vi "First Event Structure.vi"() -> ()   [LabVIEW 2015]
panel:
  out "Boolean":bool
  out "current time":timestamp
  in  "Stop":bool
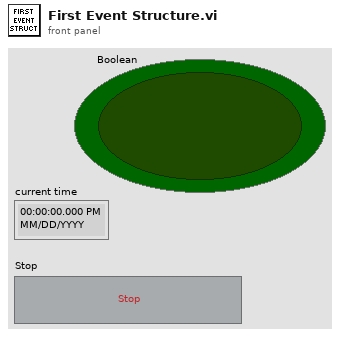
[diagram p1: front panel]
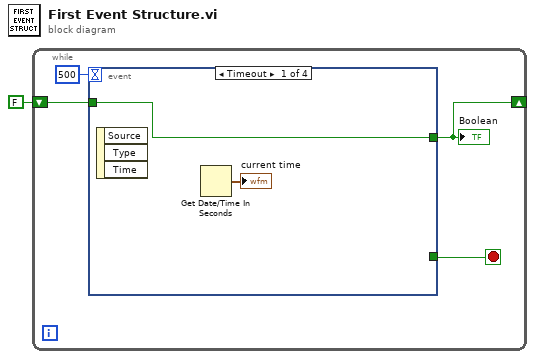
[diagram p0: block diagram]
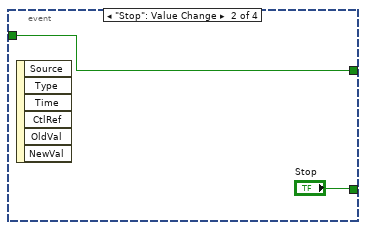
[diagram p2: hidden frame]
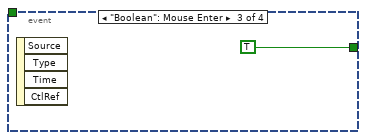
[diagram p3: hidden frame]
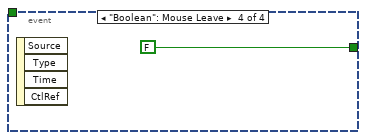
[diagram p4: hidden frame]
diagram:
  n1 = while {
    shift-right: [w3] -> _
    shift-left: FALSE ("Boolean") -> [w2]
    stop <- w4 stop-if-true
    n2 = event shown="[0] Timeout" {
      selector: _ -> [_ _ _ _]
      dyn-events: _ -> [_ _ _ _]
      timeout: 500 -> [_ _ _ _]
      tunnel: [_ "Stop" _ _] -> w4
      tunnel: [w6 w8 TRUE ("Boolean") FALSE] -> w3
      tunnel: w2 -> [w6 w8 _ _]
      event Timeout {
        n3 = event-data() -> ()  [unwired: 1 in, 3 out]
        n4 = Get Date/Time In Seconds() -> (seconds since 1Jan1904=→"current time":timestamp)
      }
      event "Stop": Value Change {
        n5 = event-data() -> ()  [unwired: 1 in, 6 out]
      }
      event "Boolean": Mouse Enter {
        n6 = event-data() -> ()  [unwired: 1 in, 4 out]
      }
      event "Boolean": Mouse Leave {
        n7 = event-data() -> ()  [unwired: 1 in, 4 out]
      }
    }
    "Boolean" <- w3
  }
